vi "Insert Ramp Rate Step.vi"(0 "VISA resource name":refnum<visa-resource-name>, 1 "Current Step Number (1)":i16=1, 2 "Wait For Event Inputs (0; 0; 0; 0)":u16[](array[ring])=[0, 0, 0, 0] items=["Don't Wait", "Wait For Off", "Wait For On"], 3 "Wait For Analog Inputs (0; 0; 0)":u16[](array[ring])=[0, 0, 0] items=["Don't Wait", "Wait For Analog Input"], 4 "Analog Input Values (32.0; 32.0; 32.0)":dbl[](array[numeric])=[32.0, 32.0, 32.0] format="%.2f", 5 "error in (no error)":errorcluster {"code" format="%.0x"}, 6 "Unit Address (1)":i16=1, 7 "Event Outputs (0; 0; 0; 0; 0; 0; 0; 0)":u16[](array[ring])=[0, 0, 0, 0, 0, 0, 0, 0] items=["Off", "On"], 8 "Wait For Event (0: No)":u16(ring) items=["No", "Yes"], 9 "Ramp Rate (0.1)":dbl=0.1 format="%.2f", 10 "Channel 1 Guarantee Soak (F: Off)":bool, 11 "Set Point Channel 1 (75.0)":dbl=75.0 format="%.2f", 13 "Channel 1 PID Set (1)":u16=1) -> (14 "VISA resource name out":refnum<visa-resource-name>, 19 "error out":errorcluster {"code" format="%.0x"})   [LabVIEW 2010]
doc: "This VI inserts Ramp Rate Step."
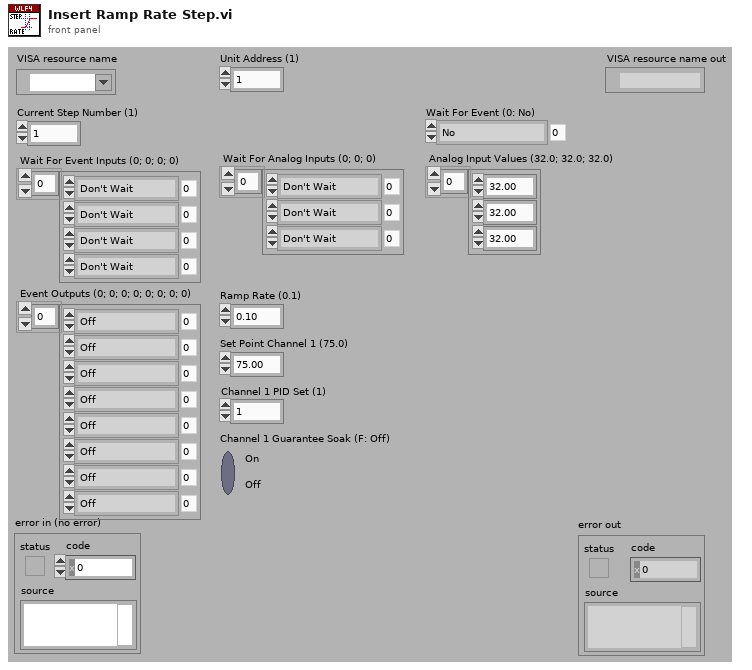
[diagram p1: front panel]
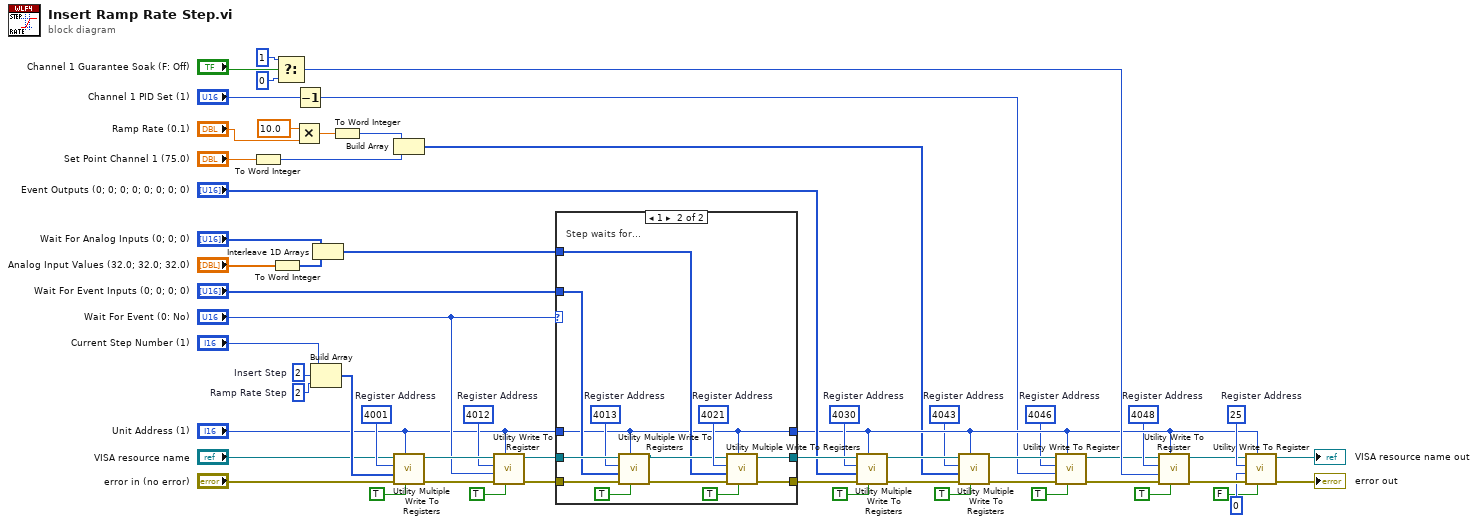
[diagram p0: block diagram]
diagram:
  w15 = u16 4048  # Register Address
  w16 = u16 4046  # Register Address
  w19 = u16 4043  # Register Address
  w20 = u16 2  # Ramp Rate Step
  w27 = u16 25  # Register Address
  w39 = u16 4030  # Register Address
  w51 = u16 4012  # Register Address
  w57 = u16 2  # Insert Step
  w59 = u16 4001  # Register Address
  n1 = To Word Integer(number="Set Point Channel 1 (75.0)") -> (16bit integer=w12:i16)
  n2 = To Word Integer(number="Analog Input Values (32.0; 32.0; 32.0)") -> (16bit integer=w44:i16[])
  n3 = Select(t=1, s="Channel 1 Guarantee Soak (F: Off)", f=0) -> (s? t:f=w28:i32)
  n4 = Multiply(x=10.0, y="Ramp Rate (0.1)") -> (x*y=w36:dbl)
  n5 = Decrement(x="Channel 1 PID Set (1)") -> (x-1=w8:u16)
  n6 = Build Array("Current Step Number (1)", w57, w20) -> (w58:u16[])
  n7 = Interleave 1D Arrays("Wait For Analog Inputs (0; 0; 0)", w44) -> (w42:u16[])
  n8 = To Word Integer(number=w36) -> (16bit integer=w11:i16)
  n9 = Build Array(w11, w12) -> (w10:i16[])
  n10 = call "Utility Multiple Write To Registers.vi"("Direct Action?"=TRUE, "Unit Address (1)"="Unit Address (1)", "error in (no error)"="error in (no error)", "Array Of Data"=w58, "Register Address (0)"=w59, "VISA resource name"="VISA resource name") -> ("error out"=w53:errorcluster, "VISA resource name out"=w52:refnum<visa-resource-name>)  [unwired: 4 in]
  n11 = call "Utility Write To Register.vi"("Direct Action?"=TRUE, "Unit Address (1)"="Unit Address (1)", "error in (no error)"=w53, "Data (0)"="Wait For Event (0: No)", "Register Address (0)"=w51, "VISA resource name"=w52) -> ("error out"=w49:errorcluster, "VISA resource name out"=w50:refnum<visa-resource-name>)  [unwired: 4 in]
  n12 = case shown="1" "Wait For Event (0: No)" {
    tunnel: w50 -> [w62 w74]
    tunnel: w49 -> [w61 w75]
    tunnel: [w61 w67] -> w41
    tunnel: [w62 w66] -> w40
    tunnel: "Unit Address (1)" -> [w60 w65]
    tunnel: [w60 w65] -> w22
    tunnel: "Wait For Event Inputs (0; 0; 0; 0)" -> [_ w72]
    tunnel: w42 -> [_ w68]
    frame 0, Default {
      # "Step does not wait"
    }
    frame 1 {
      w71 = u16 4021  # Register Address
      w73 = u16 4013  # Register Address
      # "Step waits for..."
      n13 = call "Utility Multiple Write To Registers.vi"("Direct Action?"=TRUE, "Unit Address (1)"=w65, "error in (no error)"=w75, "Array Of Data"=w72, "Register Address (0)"=w73, "VISA resource name"=w74) -> ("error out"=w70:errorcluster, "VISA resource name out"=w69:refnum<visa-resource-name>)  [unwired: 4 in]
      n14 = call "Utility Multiple Write To Registers.vi"("Direct Action?"=TRUE, "Unit Address (1)"=w65, "error in (no error)"=w70, "Array Of Data"=w68, "Register Address (0)"=w71, "VISA resource name"=w69) -> ("error out"=w67:errorcluster, "VISA resource name out"=w66:refnum<visa-resource-name>)  [unwired: 4 in]
    }
  }
  n15 = call "Utility Multiple Write To Registers.vi"("Direct Action?"=TRUE, "Unit Address (1)"=w22, "error in (no error)"=w41, "Array Of Data"="Event Outputs (0; 0; 0; 0; 0; 0; 0; 0)", "Register Address (0)"=w39, "VISA resource name"=w40) -> ("error out"=w30:errorcluster, "VISA resource name out"=w29:refnum<visa-resource-name>)  [unwired: 4 in]
  n16 = call "Utility Multiple Write To Registers.vi"("Direct Action?"=TRUE, "Unit Address (1)"=w22, "error in (no error)"=w30, "Array Of Data"=w10, "Register Address (0)"=w19, "VISA resource name"=w29) -> ("error out"=w18:errorcluster, "VISA resource name out"=w17:refnum<visa-resource-name>)  [unwired: 4 in]
  n17 = call "Utility Write To Register.vi"("Direct Action?"=TRUE, "Unit Address (1)"=w22, "error in (no error)"=w18, "Data (0)"=w8, "Register Address (0)"=w16, "VISA resource name"=w17) -> ("error out"=w14:errorcluster, "VISA resource name out"=w13:refnum<visa-resource-name>)  [unwired: 4 in]
  n18 = call "Utility Write To Register.vi"("Direct Action?"=TRUE, "Unit Address (1)"=w22, "error in (no error)"=w14, "Data (0)"=w28, "Register Address (0)"=w15, "VISA resource name"=w13) -> ("error out"=w26:errorcluster, "VISA resource name out"=w24:refnum<visa-resource-name>)  [unwired: 4 in]
  n19 = call "Utility Write To Register.vi"("Direct Action?"=FALSE, "Unit Address (1)"=w22, "error in (no error)"=w26, "Data (0)"=i16 0, "Register Address (0)"=w27, "VISA resource name"=w24) -> ("error out"=→"error out":errorcluster, "VISA resource name out"=→"VISA resource name out":refnum<visa-resource-name>)  [unwired: 4 in]
